vi "Day 02 Part 1.vi"(11 "Input":string) -> (3 "Output":dbl)   [LabVIEW 2021]
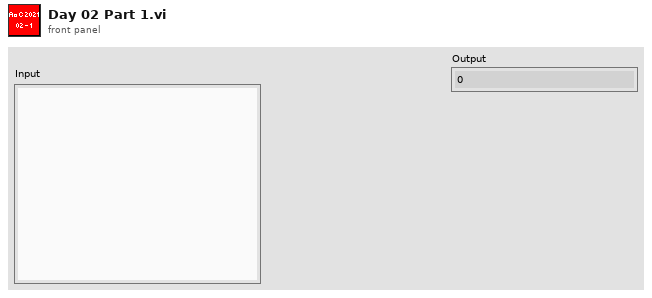
[diagram p1: front panel]
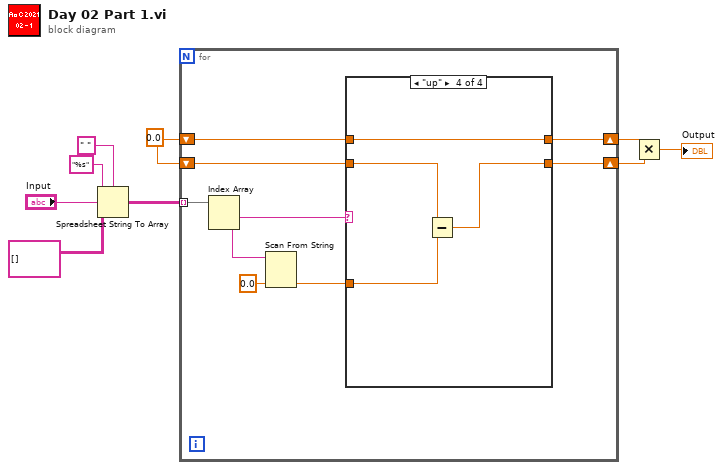
[diagram p0: block diagram]
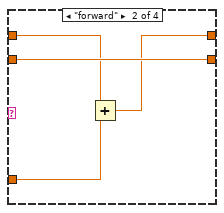
[diagram p3: hidden frame]
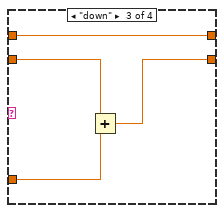
[diagram p4: hidden frame]
diagram:
  w4 = 0.0
  n1 = Spreadsheet String To Array(delimiter (Tab)=" ", format string="%s", spreadsheet string="Input", array type (2D Dbl)=string[][] []) -> (array=w5:string[][])
  n2 = for {
    tunnel: w5 -> [w18] mode=indexing
    shift-right: [w15] -> w2
    shift-left: w4 -> [w14]
    shift-right: [w10] -> w3
    shift-left: w4 -> [w16]
    n3 = Index Array(array=w18) -> (element #1=w17:string, element #2=w13:string)  [unwired: 2 in]
    n4 = Scan From String(input string=w13, default 1=0.0 ("default value 1")) -> (output 1=w12:dbl)  [unwired: 3 in, 3 out]
    n5 = case shown="\"up\"" w17 {
      tunnel: w16 -> [w19 w22 w28 w32]
      tunnel: [w20 w24 w25 w29] -> w15
      tunnel: w14 -> [w20 w24 w26 w30]
      tunnel: w12 -> [_ w23 w27 w31]
      tunnel: [w19 w21 w28 w32] -> w10
      frame Default {
      }
      frame "forward" {
        n6 = Add(x=w22, y=w23) -> (x+y=w21:dbl)
      }
      frame "down" {
        n7 = Add(x=w26, y=w27) -> (x+y=w25:dbl)
      }
      frame "up" {
        n8 = Subtract(x=w30, y=w31) -> (x-y=w29:dbl)
      }
    }
  }
  n9 = Multiply(x=w3, y=w2) -> (x*y=→"Output":dbl)
